vi "AVI-Reinitialise viewer on error.vi"(8 "error in (no error)":errorcluster, 11 "Queue in":refnum<queue>) -> (0 "error out":errorcluster)   [LabVIEW 2013]
uses:
  Typedefs/Speed Viewer States enum.ctl
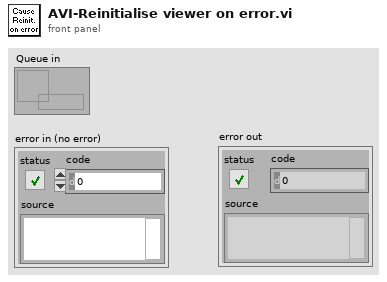
[diagram p1: front panel]
types:
  T1 = typedef "Speed Viewer States enum.ctl" = enum16{"Idle", "Initialise", "Playback", "Scroll bar event", "Speed cursor event", "Back to start", "Exit"}
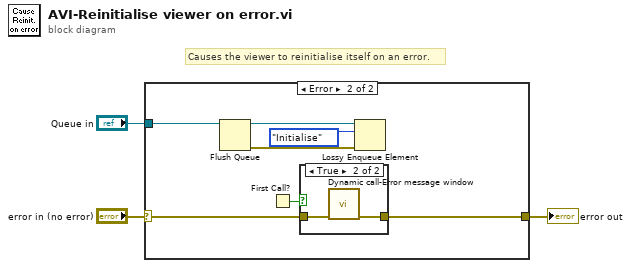
[diagram p0: block diagram]
diagram:
  # "Causes the viewer to reinitialise itself on an error."
  n1 = case shown="Error" "error in (no error)" {
    selector: "error in (no error)" -> [w4 w6]
    tunnel: "Queue in" -> [_ w9]
    tunnel: [w4 w5] -> w1
    frame No Error {
    }
    frame Error {
      n2 = Flush Queue(queue=w9) -> (queue out=w8:refnum<queue>, error out=w10:errorcluster)  [unwired: 1 in, 1 out]
      n3 = First Call?() -> (First Call?: T/F=w7:bool)
      n4 = case shown="True" w7 {
        tunnel: w6 -> [w12 w14]
        tunnel: [w12 w13] -> w5
        frame False {
        }
        frame True {
          n5 = call "Dynamic call-Error message window.vi"("error in (no error)"=w14) -> ("error out"=w13:errorcluster)  [unwired: 10 in]
        }
      }
      n6 = Lossy Enqueue Element(queue=w8, element=Speed_Viewer_States_enum."Initialise" ("States"), error in (no error)=w10) -> ()  [unwired: 4 out]
    }
  }
  "error out" <- w1
